vi "Intake Loop.vi"   [LabVIEW 2016]
uses:
  Robot Global Data.vi
types:
  T1 = typedef "Dashboard Control Data.ctl" = cluster{"Drivetrain Settings":T2, "Intake Presets ":T4, "Shooter Presets":T5, "Vision Target Packet":T8, "Auton Presets":cluster{"Start Position":dbl}, "Drivetrain Encoder Values":T9, "Drivetrain Encoder Settings":cluster{"Left Tick Constant":dbl, "Right Tick Contant":dbl, "Reset Encoders":bool, "Center Tick Constant":dbl}, "Zero Gyro":bool}
  T2 = typedef "Drivetrain Settings.ctl" = cluster{"Gyro Tolerance":dbl, "Gyro Steer PID Gains":T3, "Y Power Multiplier":dbl, "Turn Power Multiplier":dbl, "Gyro Output":dbl, "Creep Rate":dbl, "Distance Drive PID Gains":T3, "Distance Tolerance":dbl, "Distance Output":dbl, "Strafe Threshold":dbl, "Strafe Correct":bool, "Strafe Corect Tolerance":dbl, "Translate Drive PID Gains":T3, "Strafe Output":dbl, "SC Right":dbl, "SC Left":dbl, "Use Gyro":bool, "Constant Power":bool, "Strafe Power":dbl}
  T3 = typedef "PID Gains.ctl" = cluster{"proportional gain (Kc)":dbl, "integral time (Ti, min)":dbl, "derivative time (Td, min)":dbl}
  T4 = typedef "Intake Presets.ctl" = cluster{"Intake Speed ":dbl, "Outake Speed":dbl, "Current Trip Delay":dbl, "Max Current":dbl}
  T5 = typedef "Shooter Presets.ctl" = cluster{"Key Shot":cluster{"RPM ":dbl, "Hood?":bool}, "Distance Shot":cluster{"RPM":dbl, "Hood?":bool}, "RPM Tolerance":dbl, "Wheel C":dbl, "Vision Shot Presets":T6, "Hopper speed":dbl, "manuel presets":T7, "Shooter PID ":cluster{"P":dbl, "I":dbl, "D":dbl, "FF":dbl}}
  T6 = typedef "Vision Shot Presets.ctl" = cluster{"Vision Dist RPM":dbl, "Vision RPM ":dbl, "Vision Dist Hood":bool, "Vision Hood":bool, "Vision Far Dist":dbl, "is we far??":bool}
  T7 = typedef "Manual Shooter Presets.ctl" = cluster{"change delay":dbl}
  T8 = typedef "Vision Target Packet.ctl" = cluster{"Robot Center":dbl, "Center X":dbl, "Center Y":dbl, "Angle":dbl, "Distance":dbl, "Found Target?":bool}
  T9 = typedef "Drivetrain Encoder Values.ctl" = cluster{"Left Encoder":T10, "Center Encoder":T10, "Right Encoder":T10}
  T10 = typedef "Encoder Values.ctl" = cluster{"Distance":dbl, "Speed":dbl, "Tick":dbl}
  T11 = typedef "Intake Control Cluster.ctl" = cluster{"Intake Mode":T12, "Intake Auto Command":T13, "Intake Current Trip State":T14, "Fill Hopper?":bool, "Get Gear?":bool}
  T12 = typedef "Intake Modes.ctl" = enum16{"Manual", "Auto"}
  T13 = typedef "Intake Auto States.ctl" = enum16{"Outake Ball", "Idle", "Load Ball"}
  T14 = typedef "Intake Trip States.ctl" = enum16{"Normal", "Backward Tripped", "Forward Tripped"}
  T15 = typedef "Manual Command Cluster.ctl" = cluster{"Intake Power":dbl}
  T16 = typedef "WPI_MotorControlDeviceRef.ctl" = cluster{"DeviceStatus":errorcluster, "Type":T17, "PWM":cluster{"PWM Channel":T18, "DeadBand":T19}, "CAN":cluster{"Device Number":u8, "SetOutput VI Ref":variant, "GetOutput VI Ref":variant, "Enable VI Ref":variant, "Disable VI Ref":variant, "Data":variant}, "Invert":bool}
  T17 = typedef "WPI_MotorControlType.ctl" = enum16{"PWM", "CAN"}
  T18 = typedef "FPGA_DIOPWMChannel.ctl" = enum8{"PWM 0", "PWM 1", "PWM 2", "PWM 3", "PWM 4", "PWM 5", "PWM 6", "PWM 7", "PWM 8", "PWM 9", "PWM MXP 0", "PWM MXP 1", "PWM MXP 2", "PWM MXP 3", "PWM MXP 4", "PWM MXP 5", "PWM MXP 6", "PWM MXP 7", "PWM MXP 8", "PWM MXP 9", "Invalid"}
  T19 = typedef "WPI_PWMDeadband.ctl" = cluster{"Name":string, "maxPositivePwm":i32, "minPositivePwm":i32, "centerPwm":i32, "maxNegativePwm":i32, "minNegativePwm":i32, "angularRange":u16}
  T20 = typedef "Intake Status Cluster.ctl" = cluster{"Roller Power":dbl, "Intake Mode":T12, "Intake Auto State":T13, "Backward Tripped?":bool, "Forward Tripped?":bool, "Filling Hopper?":bool, "Intake Current Trip State":T14, "Getting Gear?":bool}
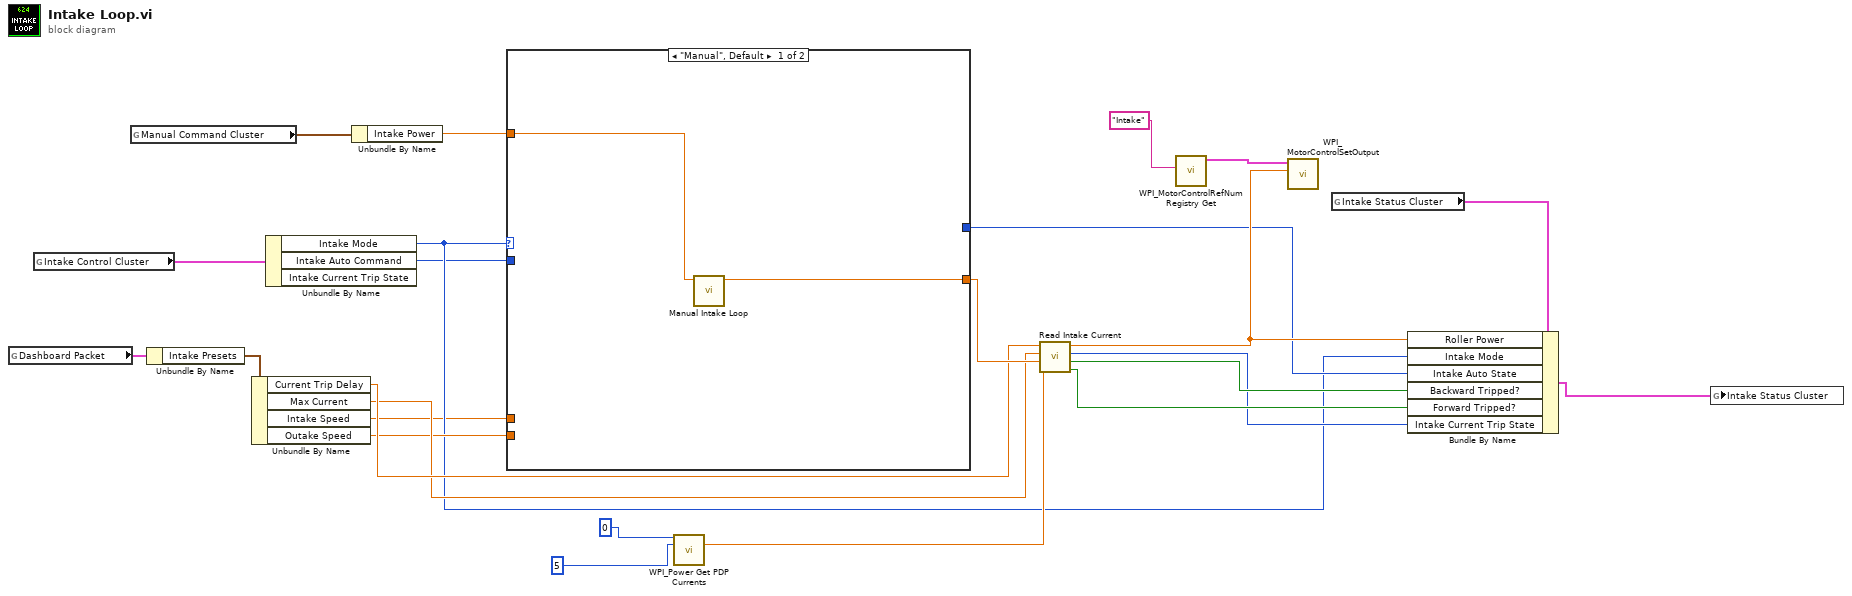
[diagram p0: block diagram]
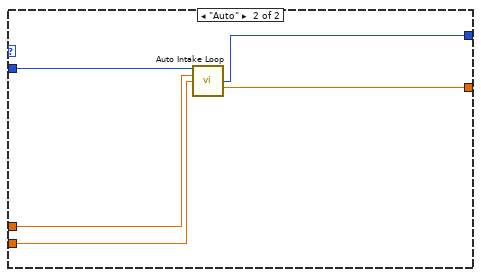
[diagram p2: hidden frame]
diagram:
  n1 = global read "Robot Global Data.vi" "Dashboard Packet"() -> (w11:T1)
  n2 = global read "Robot Global Data.vi" "Intake Control Cluster"() -> (w3:T11)
  n3 = global read "Robot Global Data.vi" "Manual Command Cluster"() -> (w21:T15)
  n4 = Unbundle By Name(w11) -> ("Intake Presets"=w12:T4)
  n5 = Unbundle By Name(w12) -> ("Current Trip Delay"=w15:dbl, "Max Current"=w14:dbl, "Intake Speed"=w1:dbl, "Outake Speed"=w13:dbl)
  n6 = Unbundle By Name(w3) -> ("Intake Mode"=w5:T12, "Intake Auto Command"=w4:T13)  [unwired: 1 out]
  n7 = Unbundle By Name(w21) -> ("Intake Power"=w22:dbl)
  n8 = case shown="\"Manual\", Default" w5 {
    tunnel: [w25 w27] -> w20
    tunnel: w22 -> [w26 _]
    tunnel: w4 -> [_ w29]
    tunnel: w1 -> [_ w31]
    tunnel: w13 -> [_ w30]
    tunnel: [_ w28] -> w6
    frame "Manual", Default {
      n9 = call "Manual Intake Loop.vi"("Intake Power"=w26) -> ("Roller Power"=w25:dbl)  [unwired: 10 in]
    }
    frame "Auto" {
      n10 = call "Auto Intake Loop.vi"("Intake Auto Commands"=w29, "Intake Power"=w31, "Outake Power"=w30) -> ("Intake State"=w28:T13, "Proposed Power"=w27:dbl)  [unwired: 11 in]
    }
  }
  n11 = call <vilib>:"WPI_Power Get PDP Currents.vi"("Power Distribution Panel (0)"=0, "PDP Channel"=5) -> ("current (A)"=w10:dbl)  [unwired: 11 in, 2 out]
  n12 = call "Read Intake Current.vi"("Current"=w10, "Proposed Power"=w20, "Max Current"=w14, "Current Trip Delay"=w15) -> ("Forward Tripped"=w19:bool, "Backward Tripped"=w18:bool, "Intake Current Trip State"=w17:T14, "Actual Power"=w16:dbl)  [unwired: 4 in]
  n13 = call <vilib>:"WPI_MotorControlRefNum Registry Get.vi"("refnum name"="Intake") -> ("MotorControlDevRef"=w23:T16)  [unwired: 9 in, 1 out]
  n14 = call <vilib>:"WPI_MotorControlSetOutput.vi"("Output"=w16, "MotorControlDevRef"=w23) -> ()  [unwired: 7 in, 3 out]
  n15 = global read "Robot Global Data.vi" "Intake Status Cluster"() -> (w2:T20)
  n16 = Bundle By Name(cluster=w2, "Roller Power"=w16, "Intake Mode"=w5, "Intake Auto State"=w6, "Backward Tripped?"=w18, "Forward Tripped?"=w19, "Intake Current Trip State"=w17) -> (w7:T20)
  n17 = global write "Robot Global Data.vi" "Intake Status Cluster"(w7) -> ()
